vi "Start Sync.vi"(8 "error in (no error)":errorcluster, 10 "current time":timestamp, 11 "gRPC Server in":refnum<class "HVC6.lvclass">) -> (0 "error out":errorcluster, 3 "gRPC Server out":refnum<class "HVC6.lvclass">)   [LabVIEW 2019, in "HVC6.lvlib" / "HVC6.lvclass"]
uses:
  HVC6.lvclass
  RPC Messages/measurementservice_QueryResponse/measurementservice_QueryResponse_Data.ctl
  RPC Messages/measurementservice_ErrorOut/measurementservice_ErrorOut_Data.ctl
  RPC Messages/measurementservice_PWMOpenSessionResponse/measurementservice_PWMOpenSessionResponse_Data.ctl
  RPC Messages/measurementservice_PWMCloseSessionResponse/measurementservice_PWMCloseSessionResponse_Data.ctl
  RPC Messages/measurementservice_PWMStartResponse/measurementservice_PWMStartResponse_Data.ctl
  Message.ctl
  <vilib>/Platform/TimedLoop/XDataNode/wakeup.ctl
  <vilib>/Platform/TimedLoop/XDataNode/XDNodeRunTimeDep.lvlib
  <vilib>/Platform/TimedLoop/XDataNode/nitl_modes.ctl
  <vilib>/Platform/TimedLoop/XDataNode/timing_clust.ctl
  <vilib>/platform/TimedLoop/XDataNode/XDataNode.xnode
  <vilib>/DAQmx/write.llb/DAQmx Write (Digital Bool 1Line 1Point).vi
  <resource>/objmgr/daqmx.rc
  State.ctl
  RPC Messages/measurementservice_PWMStopResponse/measurementservice_PWMStopResponse_Data.ctl
  <vilib>/DAQmx/create/channels.llb/DAQmx Create Channel (DO-Digital Output).vi
  RPC Messages/measurementservice_PWMModifyResponse/measurementservice_PWMModifyResponse_Data.ctl
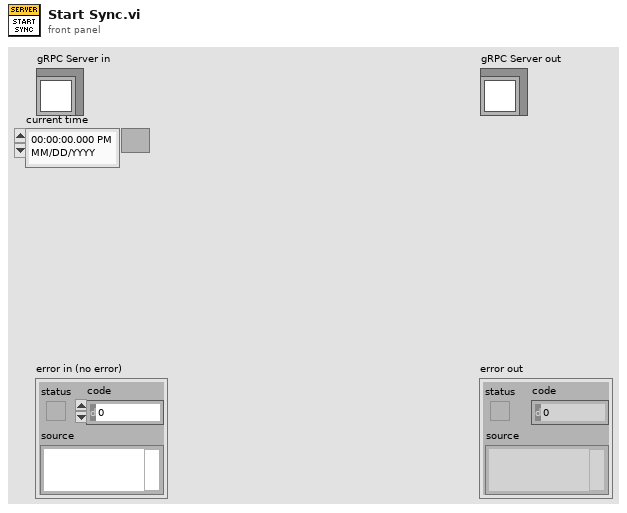
[diagram p1: front panel]
types:
  T1 = typedef "HVC6.lvlib/HVC6.lvclass/Message.ctl" = cluster{"State":T2, "PWMSession":refnum<k21>, "Period (dt)":i64}
  T2 = typedef "HVC6.lvlib/HVC6.lvclass/State.ctl" = enum16{"Start", "Update Frequency", "Stop"}
  T3 = typedef "XDNodeRunTimeDep.lvlib/timing_clust.ctl" = cluster{"Expected End [f-1]":u64, "Actual End [f-1]":u64, "Finished Late? [f-1]":bool, "Expected End [i-1]":u64, "Actual End [i-1]":u64, "Finished Late? [i-1]":bool, "Expected Start [i]":u64, "Actual Start [i]":u64, "Expected Start [f]":u64, "Actual Start [f]":u64, "Source Name":string, "Structure Name":string, "Period":i64, "Deadline":i64, "Offset":i64, "Start":i64, "Priority":i32, "Timeout":i32, "Mode":T4, "Wakeup Reason":T5, "Error":errorcluster, "Source Type":string, "Secondary Source Type":string, "Global End Time":u64, "Global Start Time":u64, "Frame Duration":u64, "Iteration Duration":u64, "Assigned CPU":i32, "I/O Scan Engine Mode":u32}
  T4 = typedef "XDNodeRunTimeDep.lvlib/nitl_modes.ctl" = enum32{"No Change", "Process missed periods, maintain original phase", "Discard missed periods, maintain original phase", "Process missed periods, ignore original phase", "Discard missed periods, ignore original phase"}
  T5 = typedef "XDNodeRunTimeDep.lvlib/wakeup.ctl" = enum32{"Normal", "Aborted", "Asynchronous wakeup", "Timing source error", "Timed loop error", "Timeout"}
  T6 = typedef "HVC6.lvlib/HVC6.lvclass/measurementservice_QueryResponse_Data.ctl" = cluster{"message":string, "status":i32}
  T7 = typedef "HVC6.lvlib/HVC6.lvclass/measurementservice_ErrorOut_Data.ctl" = cluster{"errCode":i32, "errMessage":string}
  T8 = typedef "HVC6.lvlib/HVC6.lvclass/measurementservice_PWMOpenSessionResponse_Data.ctl" = cluster{"error":T7}
  T9 = typedef "HVC6.lvlib/HVC6.lvclass/measurementservice_PWMStartResponse_Data.ctl" = cluster{"PWMInitialState":bool, "PWMInvertLines":bool, "PWMFrequency":i32, "error":T7}
  T10 = typedef "HVC6.lvlib/HVC6.lvclass/measurementservice_PWMModifyResponse_Data.ctl" = cluster{"PWMFrequency":i32, "error":T7}
  T11 = typedef "HVC6.lvlib/HVC6.lvclass/measurementservice_PWMStopResponse_Data.ctl" = cluster{"error":T7}
  T12 = typedef "HVC6.lvlib/HVC6.lvclass/measurementservice_PWMCloseSessionResponse_Data.ctl" = cluster{"error":T7}
  T13 = typedef "HVC6.lvlib/HVC6.lvclass/Server gRPC UEs.ctl" = cluster{"Invoke gRPC UE":refnum<user-event>, "Query gRPC UE":refnum<user-event>, "Register gRPC UE":refnum<user-event>, "OpenPWMSession gRPC UE":refnum<user-event>, "StartPWM gRPC UE":refnum<user-event>, "ModifyPWM gRPC UE":refnum<user-event>, "StopPWM gRPC UE":refnum<user-event>, "ClosePWMSession gRPC UE":refnum<user-event>}
  T14 = typedef "HVC6.lvlib/gprc-lvsupport.lvlib/grpcId.ctl" = u64
  T15 = typedef "HVC6.lvlib/HVC6.lvclass/measurementservice_QueryRequest_Data.ctl" = cluster{"query":string}
  T16 = typedef "HVC6.lvlib/HVC6.lvclass/measurementservice_PWMOpenSessionRequest_Data.ctl" = cluster{"PWMlines":string}
  T17 = typedef "HVC6.lvlib/HVC6.lvclass/measurementservice_PWMStartRequest_Data.ctl" = cluster{"PWMInitialState":bool, "PWMInvertLines":bool, "PWMFrequency":i32}
  T18 = typedef "HVC6.lvlib/HVC6.lvclass/measurementservice_PWMModifyRequest_Data.ctl" = cluster{"PWMFrequency":i32}
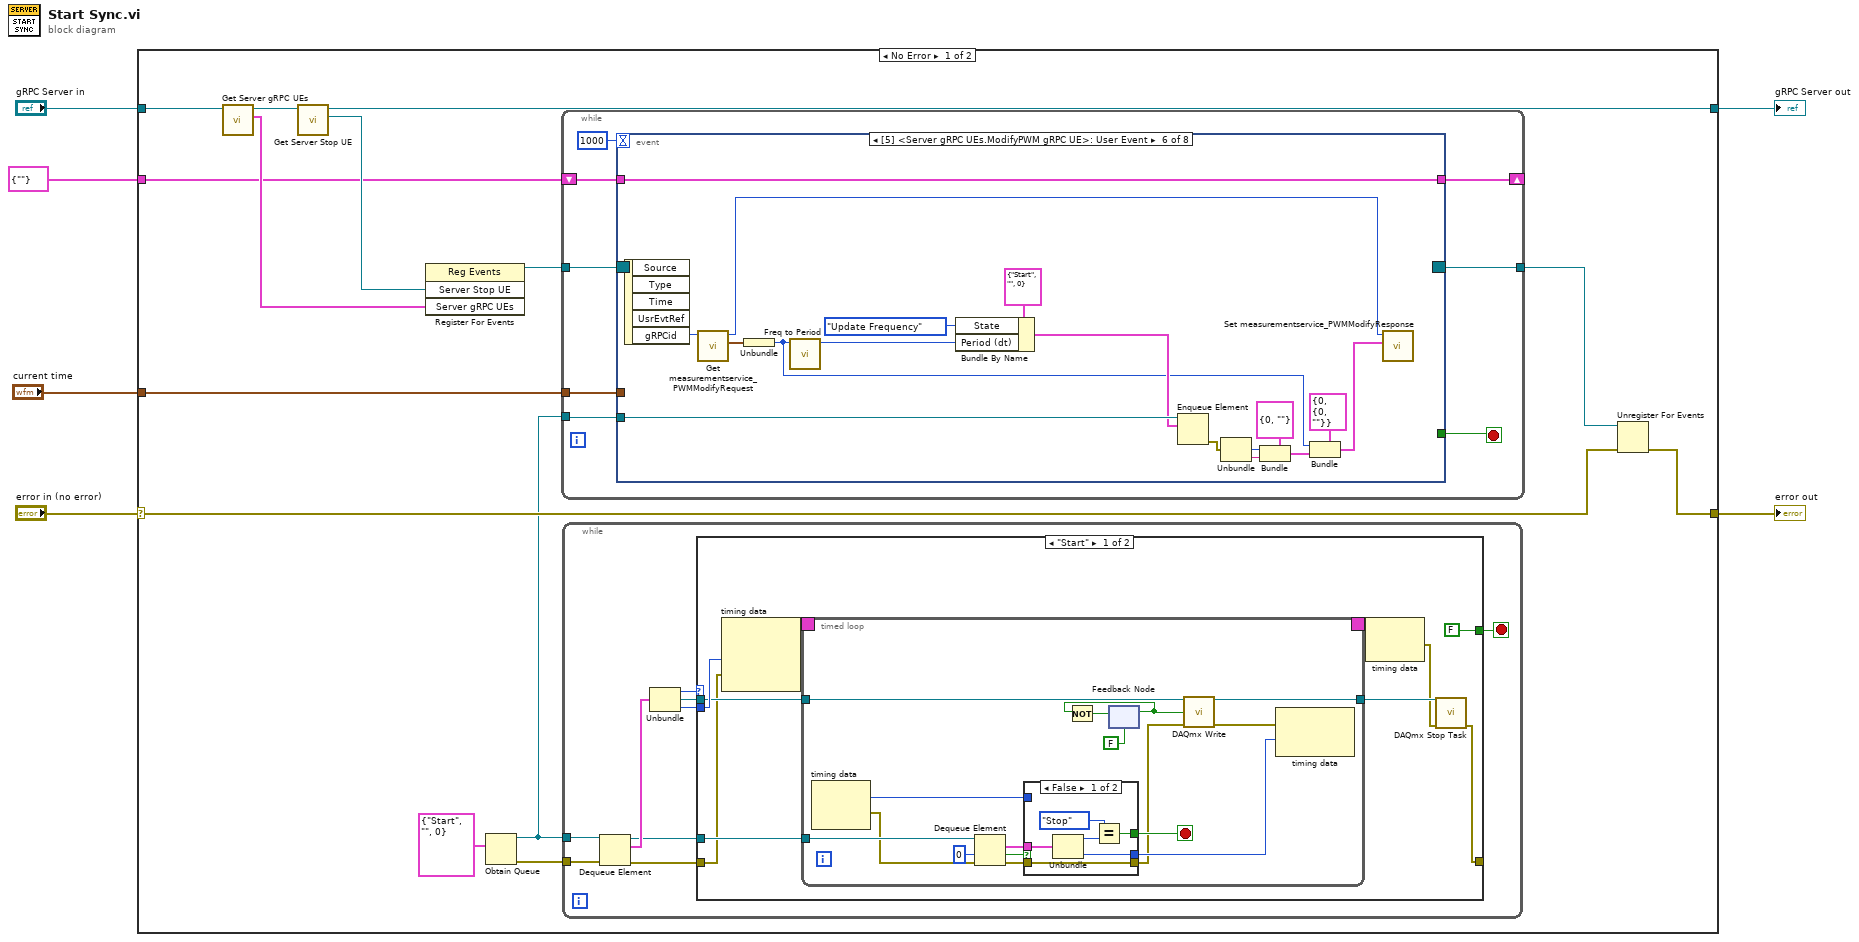
[diagram p0: block diagram]
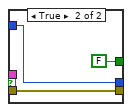
[diagram p2: hidden frame]
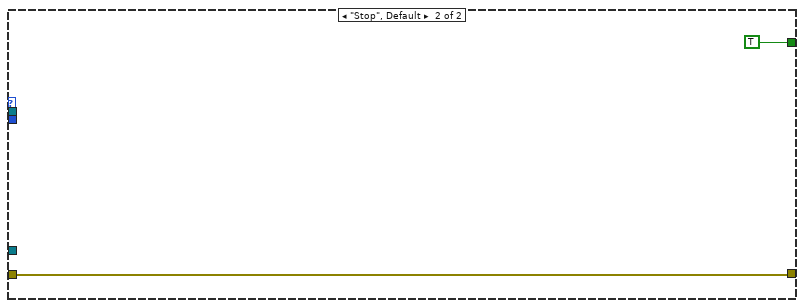
[diagram p3: hidden frame]
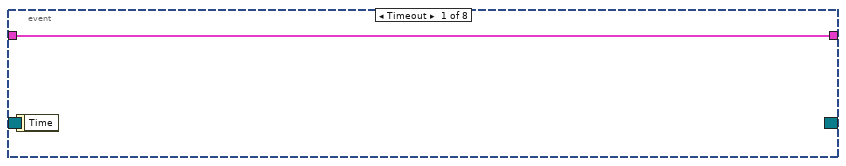
[diagram p4: hidden frame]
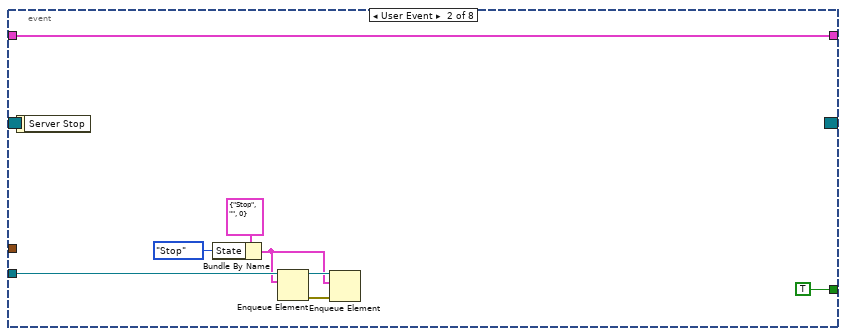
[diagram p5: hidden frame]
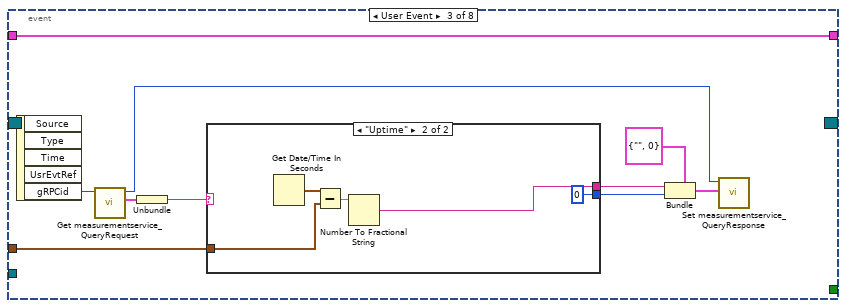
[diagram p6: hidden frame]
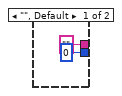
[diagram p7: hidden frame]
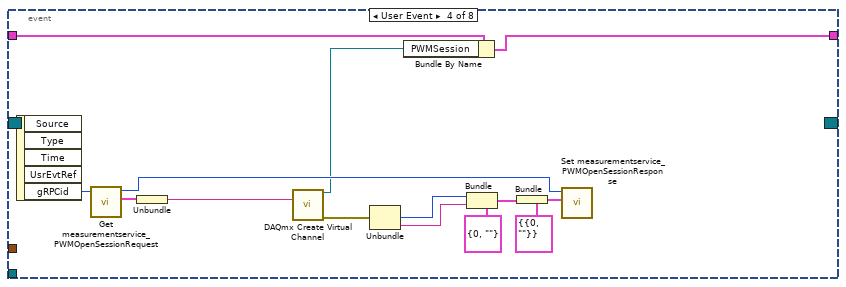
[diagram p8: hidden frame]
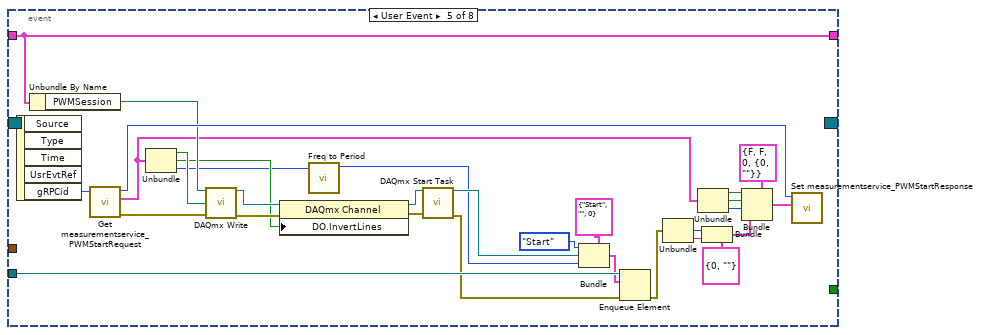
[diagram p9: hidden frame]
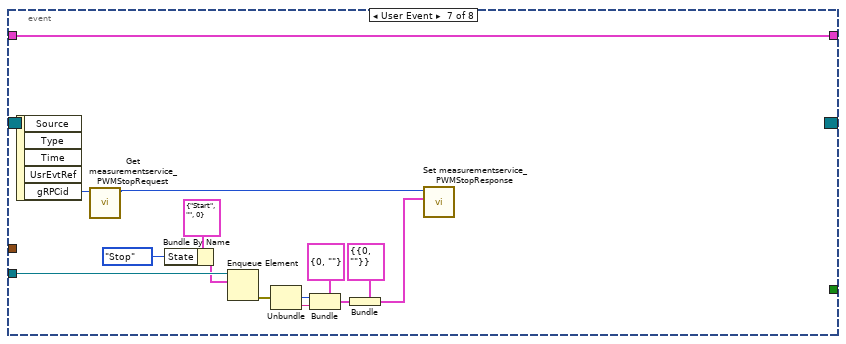
[diagram p10: hidden frame]
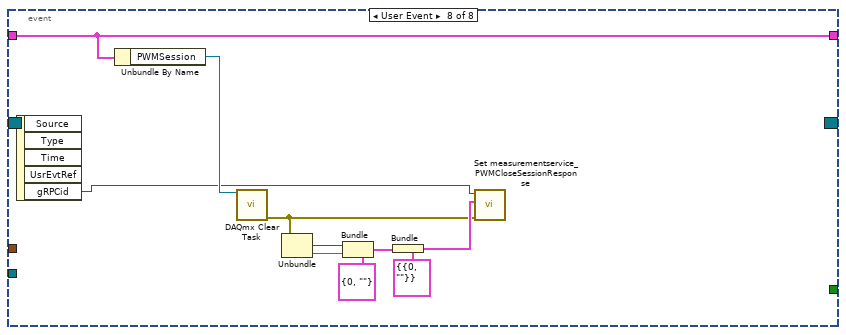
[diagram p11: hidden frame]
diagram:
  n1 = case shown="No Error" "error in (no error)" {
    selector: "error in (no error)" -> [w13 w200]
    tunnel: [w12 w200] -> w5
    tunnel: [w16 w199] -> w3
    tunnel: "gRPC Server in" -> [w20 w199]
    tunnel: "current time" -> [w11 _]
    tunnel: cluster{"PWMSession":refnum<k21>} {"PWMSession"=""} -> [w10 _]
    frame No Error {
      n2 = call "Get Server gRPC UEs.vi"("OOP Server in"=w20) -> ("Server gRPC UEs"=w17:T13, "OOP Server out"=w19:refnum<class "HVC6.lvclass">)  [unwired: 9 in]
      n3 = call "Get Server Stop UE.vi"("OOP Server in"=w19) -> ("Server Stop UE"=w18:refnum<user-event>, "OOP Server out"=w16:refnum<class "HVC6.lvclass">)  [unwired: 9 in]
      n4 = register-events(w18, w17) -> (reference out=w15:refnum<event-registration>)  [unwired: 2 in, 1 out]
      n5 = Obtain Queue(element data type=T1 {"State"=enum."Start", "PWMSession"="", "Period (dt)"=0} ("Message Cluster")) -> (queue out=w7:refnum<queue>, error out=w8:errorcluster)  [unwired: 4 in, 1 out]
      n6 = while {
        tunnel: w15 -> [w87]
        tunnel: [w85] -> w14
        tunnel: w11 -> [w83]
        shift-right: [w81] -> _
        shift-left: w10 -> [w82]
        tunnel: w7 -> [w80]
        stop <- w86 stop-if-true
        n7 = event "RPC Methods Event Structure" shown="[5] <Server gRPC UEs.ModifyPWM gRPC UE>: User Event" {
          selector: w87 -> [_ _ _ _ _ _ _ _]
          dyn-events: [_ _ _ _ _ _ _ _] -> w85
          timeout: 1000 -> [_ _ _ _ _ _ _ _]
          tunnel: [_ TRUE _ _ _ _ _ _] -> w86
          tunnel: w83 -> [_ _ w98 _ _ _ _ _]
          tunnel: w82 -> [w88 w95 w97 w115 w128 w167 w181 w196]
          tunnel: [w88 w95 w97 w114 w128 w167 w181 w196] -> w81
          tunnel: w80 -> [_ w94 _ _ w153 w174 w188 _]
          event Timeout {
            n8 = event-data() -> ()  [unwired: 1 in, 1 out]
          }
          event User Event {
            n9 = event-data() -> ()  [unwired: 1 in, 1 out]
            n10 = Bundle By Name(cluster=T1 {"State"=enum."Stop", "PWMSession"="", "Period (dt)"=0} ("element"), "State"=State."Stop") -> (w89:T1)
            n11 = Enqueue Element(queue=w94, element=w89) -> (queue out=w90:refnum<queue>, error out=w91:errorcluster)  [unwired: 2 in, 1 out]
            n12 = Enqueue Element(queue=w90, element=w89, error in (no error)=w91) -> ()  [unwired: 1 in, 3 out]
          }
          event User Event {
            n13 = event-data() -> ("gRPCid"=w106:T14)  [unwired: 1 in, 4 out]
            n14 = call "Get measurementservice_QueryRequest.vi"("gRPCid"=w106) -> ("Message Data"=w105:T15, "gRPCid out"=w102:T14)  [unwired: 8 in, 1 out]
            n15 = Unbundle(w105) -> ("query"=w101:string)
            n16 = case shown="\"Uptime\"" w101 {
              tunnel: [0 ("status") 0 ("status")] -> w100
              tunnel: ["" ("message") w110] -> w99
              tunnel: w98 -> [_ w112]
              frame "", Default {
              }
              frame "Uptime" {
                n17 = Get Date/Time In Seconds() -> (seconds since 1Jan1904=w113:timestamp)
                n18 = Subtract(x=w113, y=w112) -> (x-y=w111:dbl)
                n19 = Number To Fractional String(number=w111) -> (F-format string=w110:string)  [unwired: 3 in]
              }
            }
            n20 = Bundle(cluster=T6 {"message"="", "status"=0} ("Message Data"), "message"=w99, "status"=w100) -> (w103:T6)
            n21 = call "Set measurementservice_QueryResponse.vi"("Message Data"=w103, "gRPCid"=w102) -> ()  [unwired: 9 in, 1 out]
          }
          event User Event {
            n22 = event-data() -> ("gRPCid"=w127:T14)  [unwired: 1 in, 4 out]
            n23 = call "Get measurementservice_PWMOpenSessionRequest.vi"("gRPCid"=w127) -> ("Message Data"=w126:T16, "gRPCid out"=w123:T14)  [unwired: 8 in, 1 out]
            n24 = Unbundle(w126) -> ("PWMlines"=w120:string)
            n25 = call-poly <vilib>:"DAQmx Create Virtual Channel.vi"("lines"=w120) -> ("task out"=w116:refnum<k21>, "error out"=w119:errorcluster)  [unwired: 13 in]
            n26 = Unbundle(w119) -> ("code"=w118:i32, "source"=w117:string)  [unwired: 1 out]
            n27 = Bundle By Name(cluster=w115, "PWMSession"=w116) -> (w114:cluster{"PWMSession":refnum<k21>})
            n28 = Bundle(cluster=T7 {"errCode"=0, "errMessage"=""} ("error"), "errCode"=w118, "errMessage"=w117) -> (w121:T7)
            n29 = Bundle(cluster=T8 {"error"={"errCode"=0, "errMessage"=""}} ("measurementservice_PWMOpenSessionResponse_Data"), "error"=w121) -> (w124:T8)
            n30 = call "Set measurementservice_PWMOpenSessionResponse.vi"("Message Data"=w124, "gRPCid"=w123) -> ()  [unwired: 9 in, 1 out]
          }
          event User Event {
            n31 = event-data() -> ("gRPCid"=w157:T14)  [unwired: 1 in, 4 out]
            n32 = Unbundle By Name(w128) -> ("PWMSession"=w142:refnum<k21>)
            n33 = call "Get measurementservice_PWMStartRequest.vi"("gRPCid"=w157) -> ("error out"=w139:errorcluster, "Message Data"=w141:T17, "gRPCid out"=w154:T14)  [unwired: 8 in]
            n34 = Unbundle(w141) -> ("PWMInitialState"=w140:bool, "PWMInvertLines"=w136:bool, "PWMFrequency"=w132:i32)
            n35 = call-poly <vilib>:"DAQmx Write.vi"("task/channels in"=w142, "data"=w140, "error in"=w139) -> ("task out"=w138:refnum<k21>, "error out"=w137:errorcluster)  [unwired: 10 in, 1 out]
            n36 = property class="DAQmx Channel"(reference=w138, error in=w137, "DO.InvertLines"=w136) -> (reference out=w135:refnum<k21>, error out=w134:errorcluster)
            n37 = call "Freq to Period.vi"("PWMFrequency"=w132) -> ("Period (dt)"=w130:i64)  [unwired: 10 in]
            n38 = call <vilib>:"DAQmx Start Task.vi"("task/channels in"=w135, "error in"=w134) -> ("task out"=w131:refnum<k21>, "error out"=w133:errorcluster)  [unwired: 12 in]
            n39 = Bundle(cluster=T1 {"State"=enum."Start", "PWMSession"="", "Period (dt)"=0} ("element"), "State"=State."Start", "PWMSession"=w131, "Period (dt)"=w130) -> (w148:T1)
            n40 = Enqueue Element(queue=w153, element=w148, error in (no error)=w133) -> (error out=w145:errorcluster)  [unwired: 1 in, 2 out]
            n41 = Unbundle(w145) -> ("code"=w144:i32, "source"=w143:string)  [unwired: 1 out]
            n42 = Unbundle(w141) -> ("PWMInitialState"=w152:bool, "PWMInvertLines"=w151:bool, "PWMFrequency"=w149:i32)
            n43 = Bundle(cluster=T7 {"errCode"=0, "errMessage"=""} ("error"), "errCode"=w144, "errMessage"=w143) -> (w146:T7)
            n44 = Bundle(cluster=T9 {"PWMInitialState"=FALSE, "PWMInvertLines"=FALSE, "PWMFrequency"=0, "error"={"errCode"=0, "errMessage"=""}} ("measurementservice_PWMStartResponse_Data"), "PWMInitialState"=w152, "PWMInvertLines"=w151, "PWMFrequency"=w149, "error"=w146) -> (w155:T9)
            n45 = call "Set measurementservice_PWMStartResponse.vi"("Message Data"=w155, "gRPCid"=w154) -> ()  [unwired: 9 in, 1 out]
          }
          event User Event {
            n46 = event-data() -> ("gRPCid"=w164:T14)  [unwired: 1 in, 4 out]
            n47 = call "Get measurementservice_PWMModifyRequest.vi"("gRPCid"=w164) -> ("Message Data"=w162:T18, "gRPCid out"=w163:T14)  [unwired: 8 in, 1 out]
            n48 = Unbundle(w162) -> ("PWMFrequency"=w158:i32)
            n49 = call "Freq to Period.vi"("PWMFrequency"=w158) -> ("Period (dt)"=w159:i64)  [unwired: 10 in]
            n50 = Bundle By Name(cluster=T1 {"State"=enum."Start", "PWMSession"="", "Period (dt)"=0} ("element"), "State"=State."Update Frequency", "Period (dt)"=w159) -> (w172:T1)
            n51 = Enqueue Element(queue=w174, element=w172) -> (error out=w171:errorcluster)  [unwired: 2 in, 2 out]
            n52 = Unbundle(w171) -> ("code"=w170:i32, "source"=w169:string)  [unwired: 1 out]
            n53 = Bundle(cluster=T7 {"errCode"=0, "errMessage"=""} ("error"), "errCode"=w170, "errMessage"=w169) -> (w160:T7)
            n54 = Bundle(cluster=T10 {"PWMFrequency"=0, "error"={"errCode"=0, "errMessage"=""}} ("measurementservice_PWMModifyResponse_Data"), "PWMFrequency"=w158, "error"=w160) -> (w166:T10)
            n55 = call "Set measurementservice_PWMModifyResponse.vi"("Message Data"=w166, "gRPCid"=w163) -> ()  [unwired: 9 in, 1 out]
          }
          event User Event {
            n56 = event-data() -> ("gRPCid"=w180:T14)  [unwired: 1 in, 4 out]
            n57 = call "Get measurementservice_PWMStopRequest.vi"("gRPCid"=w180) -> ("gRPCid out"=w179:T14)  [unwired: 8 in, 2 out]
            n58 = Bundle By Name(cluster=T1 {"State"=enum."Start", "PWMSession"="", "Period (dt)"=0} ("element"), "State"=State."Stop") -> (w186:T1)
            n59 = Enqueue Element(queue=w188, element=w186) -> (error out=w185:errorcluster)  [unwired: 2 in, 2 out]
            n60 = Unbundle(w185) -> ("code"=w184:i32, "source"=w183:string)  [unwired: 1 out]
            n61 = Bundle(cluster=T7 {"errCode"=0, "errMessage"=""} ("error"), "errCode"=w184, "errMessage"=w183) -> (w176:T7)
            n62 = Bundle(cluster=T11 {"error"={"errCode"=0, "errMessage"=""}} ("Message Data"), "error"=w176) -> (w175:T11)
            n63 = call "Set measurementservice_PWMStopResponse.vi"("Message Data"=w175, "gRPCid"=w179) -> ()  [unwired: 9 in, 1 out]
          }
          event User Event {
            n64 = event-data() -> ("gRPCid"=w194:T14)  [unwired: 1 in, 4 out]
            n65 = Unbundle By Name(w196) -> ("PWMSession"=w195:refnum<k21>)
            n66 = call <vilib>:"DAQmx Clear Task.vi"("task in"=w195) -> ("error out"=w189:errorcluster)  [unwired: 14 in]
            n67 = Unbundle(w189) -> ("code"=w198:i32, "source"=w197:string)  [unwired: 1 out]
            n68 = Bundle(cluster=T7 {"errCode"=0, "errMessage"=""} ("error"), "errCode"=w198, "errMessage"=w197) -> (w190:T7)
            n69 = Bundle(cluster=T12 {"error"={"errCode"=0, "errMessage"=""}} ("Message Data"), "error"=w190) -> (w192:T12)
            n70 = call "Set measurementservice_PWMCloseSessionResponse.vi"("error in (no error)"=w189, "Message Data"=w192, "gRPCid"=w194) -> ()  [unwired: 8 in, 1 out]
          }
        }
      }
      n71 = while {
        tunnel: w8 -> [w29]
        tunnel: w7 -> [w28]
        stop <- w23 stop-if-true
        n72 = Dequeue Element(queue=w28, error in (no error)=w29) -> (queue out=w26:refnum<queue>, element=w27:T1, error out=w21:errorcluster)  [unwired: 1 in, 1 out]
        n73 = Unbundle(w27) -> ("State"=w24:T2, "PWMSession"=w25:refnum<k21>, "Period (dt)"=w22:i64)
        n74 = case shown="\"Start\"" w24 {
          tunnel: w26 -> [w37 _]
          tunnel: w25 -> [w34 _]
          tunnel: [FALSE TRUE] -> w23
          tunnel: w22 -> [w35 _]
          tunnel: w21 -> [w33 w78]
          tunnel: [w30 w78] -> _
          frame "Start" {
            n75 = node-c288(w35, w33) -> (w39:T3)  [unwired: 1 in]
            n76 = timed-loop {
              timing: w39 -> [_]
              timing-out: [_] -> w38
              tunnel: [w54] -> w32
              tunnel: w37 -> [w50]
              tunnel: w34 -> [w46]
              stop <- w44 stop-if-true
              n77 = node-c288() -> (w41:i64, w49:errorcluster)  [unwired: 1 in]
              n78 = Dequeue Element(queue=w50, timeout in ms (-1)=0, error in (no error)=w49) -> (element=w48:T1, timed out?=w42:bool, error out=w43:errorcluster)  [unwired: 1 out]
              n79 = case shown="False" w42 {
                tunnel: w48 -> [w61 _]
                tunnel: [w60 w63] -> w45
                tunnel: [w57 FALSE] -> w44
                tunnel: w43 -> [w56 w62]
                tunnel: [w56 w62] -> w40
                tunnel: w41 -> [_ w63]
                frame False {
                  n80 = Unbundle(w61) -> ("State"=w58:T2, "Period (dt)"=w60:i64)  [unwired: 1 out]
                  n81 = Equal?(x=State."Stop" ("State"), y=w58) -> (x = y?=w57:bool)
                }
                frame True {
                }
              }
              n82 = feedback #1(FALSE) -> (w52:bool)
              n83 = Not(x=w52) -> (.not. x?=w51:bool)
              n84 = feedback-in #1(w51) -> ()
              n85 = call-poly <vilib>:"DAQmx Write.vi"("task/channels in"=w46, "data"=w52, "error in"=w40) -> ("task out"=w54:refnum<k21>, "error out"=w55:errorcluster)  [unwired: 10 in, 1 out]
              n86 = node-c288(w55, w45) -> ()  [unwired: 1 out]
            }
            n87 = node-c288(w38) -> (w31:errorcluster)
            n88 = call <vilib>:"DAQmx Stop Task.vi"("task/channels in"=w32, "error in"=w31) -> ("error out"=w30:errorcluster)  [unwired: 12 in, 1 out]
          }
          frame "Stop", Default {
          }
        }
      }
      n89 = Unregister For Events(event registration refnum=w14, error in=w13) -> (error out=w12:errorcluster)
    }
    frame Error {
    }
  }
  "error out" <- w5
  "gRPC Server out" <- w3
